vi "Launch Root Model.vi"(8 "error in (no error)":errorcluster, 11 "PublishingViewModel In":refnum<class "PublishingViewModel.lvclass">) -> (0 "error out":errorcluster, 3 "PublishingViewModel Out":refnum<class "PublishingViewModel.lvclass">)   [LabVIEW 2017, in "TestPubSubRouting.lvlib" / "PublishingViewModel.lvclass"]
doc: "<License>\nCopyright © 2017 Composed Systems, LLC | All rights reserved\nwww.composed.io\n\nAuthor: Ethan Stern <ethan.stern@composed.io>\n\nThis software is provided \"AS IS\" WITHOUT WARRANTIES, either express or implied, AND IS FOR EDUCATIONAL PURPOSES ONLY.\n</License>"
uses:
  PublishingViewModel.lvclass
  gpm_packages/@cs/mva-viewable/Source/IViewModel/IViewModel/IViewModel.lvclass
  C:/Git/mva-framework/Source/Framework/IViewModel/IViewModel/IViewModel.lvclass
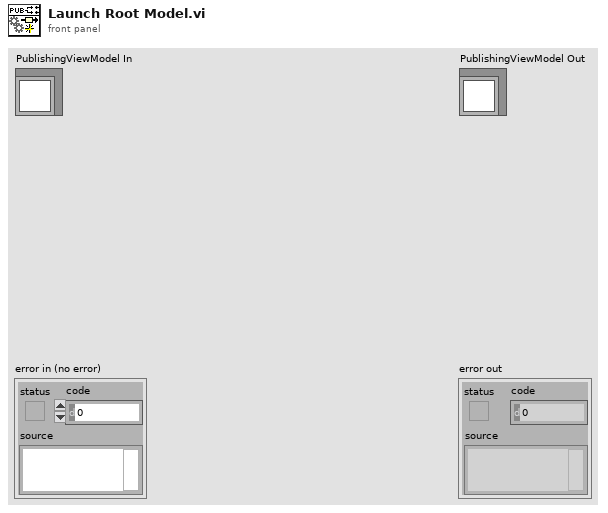
[diagram p1: front panel]
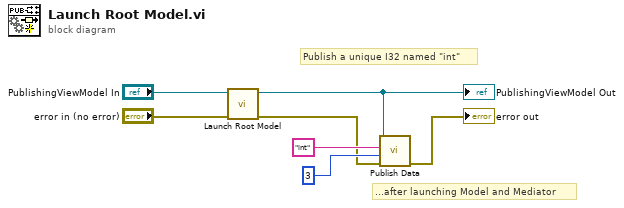
[diagram p0: block diagram]
diagram:
  # "...after launching Model and Mediator"
  # "Publish a unique I32 named \"int\""
  n1 = call-parent "Launch Root Model.vi"("error in (no error)"="error in (no error)", "IViewModel In"="PublishingViewModel In") -> ("error out"=w3:errorcluster, "IViewModel Out"=w2:refnum<class "PublishingViewModel.lvclass">)  [unwired: 8 in]
  "PublishingViewModel Out" <- w2
  n2 = call "Publish Data.vi"("error in (no error)"=w3, "Data to Publish"=3, "Datum Name"="int", "IViewModel In"=w2) -> ("error out"=→"error out":errorcluster)  [unwired: 6 in, 1 out]
